vi "Host.vi"() -> ()   [LabVIEW 2015]
panel:
  in  "stop":bool
  out "error out":errorcluster
  out "Waveform Chart":waveform(dbl)(graph)
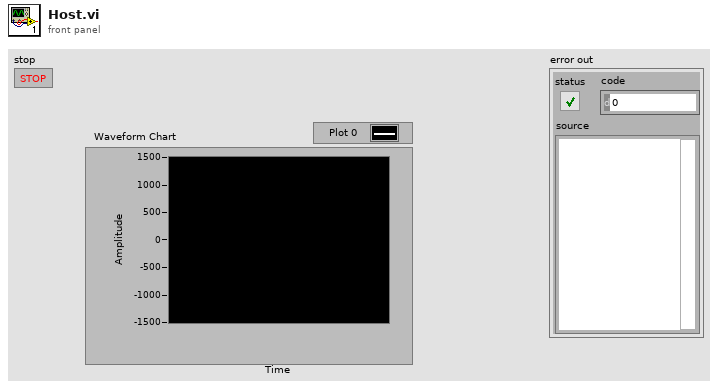
[diagram p1: front panel]
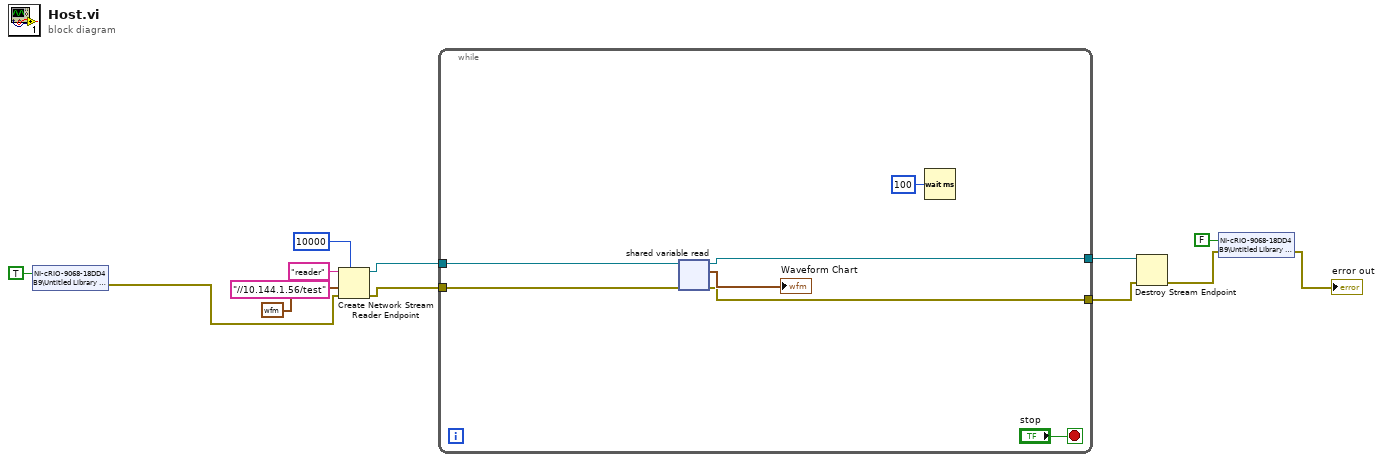
[diagram p0: block diagram]
diagram:
  n1 = shared-variable "NI-cRIO-9068-18DD4B9\\Untitled Library 1.lvlib\\signal"(TRUE ("signal")) -> (error out=w1:errorcluster)  [unwired: 1 in]
  n2 = Create Network Stream Reader Endpoint(7:10000 ("reader buffer size"), 8:w1, 9:waveform(dbl) {"t0"=timestamp(0 s since 1904-01-01), "dt"=1.0, "Y"=[]} ("Waveform"), 10:"//10.144.1.56/test" ("writer url"), 11:"reader" ("reader name")) -> (0:w10:errorcluster, 3:w9:refnum<k21>)  [unwired: 2 in]
  n3 = while {
    tunnel: w10 -> [w20]
    tunnel: w9 -> [w19]
    tunnel: [w16] -> w8
    tunnel: [w15] -> w7
    stop <- "stop" stop-if-true
    n4 = shared-variable-read(w19, w20) -> (w16:refnum<k21>, w15:errorcluster, →"Waveform Chart":waveform(dbl))  [unwired: 1 in, 1 out]
    n5 = Wait (ms)(milliseconds to wait=u32 100) -> ()  [unwired: 1 out]
  }
  n6 = Destroy Stream Endpoint(8:w7, 11:w8) -> (0:w3:errorcluster)
  n7 = shared-variable "NI-cRIO-9068-18DD4B9\\Untitled Library 1.lvlib\\signal"(FALSE ("signal"), error in=w3) -> (error out=→"error out":errorcluster)
